vi "encoder_io_read.vi"(2 "PhaseB":refnum<k21>="ConnectorA/DIO12", 3 "PhaseA":refnum<k21>="ConnectorA/DIO11") -> (0 "PhaseB":bool, 1 "PhaseA":bool)   [LabVIEW 2019]
uses:
  <vilib>/rvi/eio/common/nirviEmuTemplateMethod_errors.vi
  <vilib>/eio/EIOMethodNode/EIOMethodNode.xnode
  <vilib>/eio/EIONode/EIONode.xnode
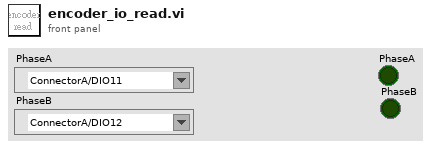
[diagram p1: front panel]
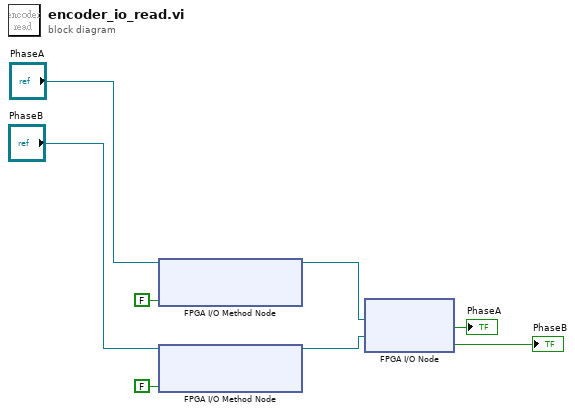
[diagram p0: block diagram]
diagram:
  n1 = xnode "FPGA I/O Method Node"("FPGA I/O In"="PhaseA", "Enable"=FALSE) -> ("FPGA I/O Out"=w2:refnum<k21>)
  n2 = xnode "FPGA I/O Method Node"("FPGA I/O In"="PhaseB", "Enable"=FALSE) -> ("FPGA I/O Out"=w1:refnum<k21>)
  n3 = xnode "FPGA I/O Node"("FPGA I/O In"=w2, "FPGA I/O In"=w1) -> ("I/O Item"=→"PhaseA":bool, "I/O Item"=→"PhaseB":bool)  [unwired: 2 out]
